vi "generate header file from param cluster.vi"(8 "output cluster":T1, 11 "header path (full)":path=path "C:/Users/QDM2exp/Documents/PK/LabView dev/pk camera stuff") -> ()   [LabVIEW 2018]
uses:
  <vilib>/Utility/file.llb/Write Delimited Spreadsheet (string).vi
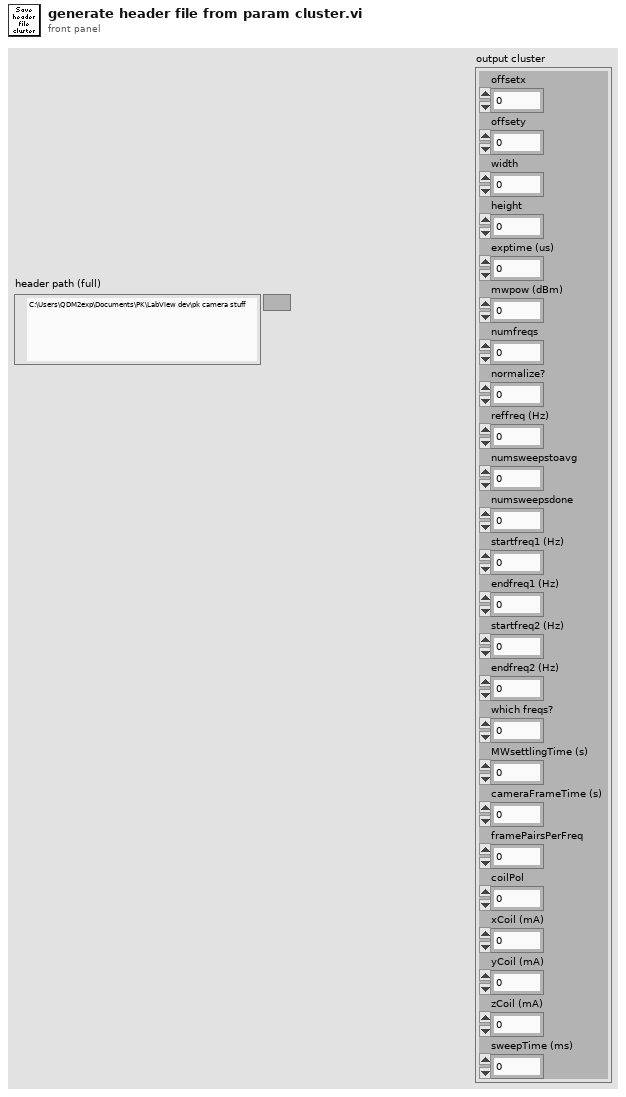
[diagram p1: front panel]
types:
  T1 = cluster{"offsetx":i64, "offsety":i64, "width":i64, "height":i64, "exptime (us)":dbl, "mwpow (dBm)":dbl, "numfreqs":i32, "normalize?":i32, "reffreq (Hz)":dbl, "numsweepstoavg":i32, "numsweepsdone":i32, "startfreq1 (Hz)":dbl, "endfreq1 (Hz)":dbl, "startfreq2 (Hz)":dbl, "endfreq2 (Hz)":dbl, "which freqs?":i32, "MWsettlingTime (s)":dbl, "cameraFrameTime (s)":dbl, "framePairsPerFreq":i32, "coilPol":i32, "xCoil (mA)":dbl, "yCoil (mA)":dbl, "zCoil (mA)":dbl, "sweepTime (ms)":i32}
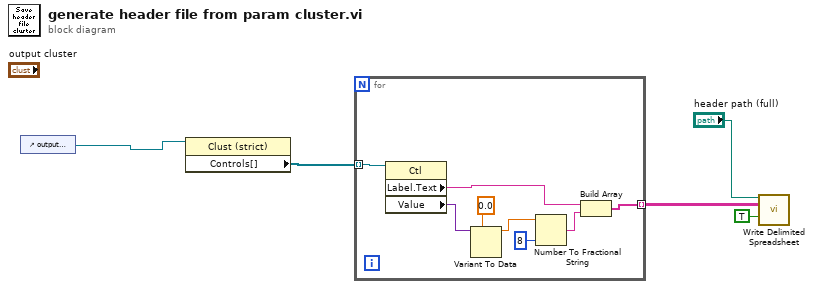
[diagram p0: block diagram]
diagram:
  n1 = control-ref of="output cluster"() -> (w1:refnum<vi>)
  n2 = property class="Clust (strict)"(reference=w1) -> ("Controls[]"=w5:refnum<vi>[])  [unwired: 1 in, 2 out]
  n3 = for {
    tunnel: w5 -> [w13] mode=indexing
    tunnel: [w7] -> w4 mode=indexing
    n4 = property class="Ctl"(reference=w13) -> ("Label.Text"=w8:string, "Value"=w12:variant)  [unwired: 1 in, 2 out]
    n5 = Variant To Data(type=0.0, Variant=w12) -> (data=w10:dbl)  [unwired: 1 in, 1 out]
    n6 = Number To Fractional String(number=w10, precision (6)=i16 8) -> (F-format string=w9:string)  [unwired: 2 in]
    n7 = Build Array(w8, w9) -> (w7:string[])
  }
  n8 = call-poly <vilib>:"Write Delimited Spreadsheet.vi"("file path (dialog if empty)"="header path (full)", "2D data"=w4, "append to file? (new file:F)"=TRUE) -> ()  [unwired: 11 in, 2 out]
